vi "rsidr_core_global.vi"() -> ()   [LabVIEW 2020, in "Rohde&Schwarz CMWXP NR FR1 Measurement.lvlib"] (continued)
measured list mode segments.\n\nReturn values:  \n<Reliability>\n decimal\n\n<TimingError>\n float\nComma-separated list of values, one per measured segment\nDefault unit:  Ts (basic time unit)\n\nAvailable Repeated Capabilities:\ninstance: i0, i1, i2, i3, i4, i5, i6, i7, i8, i9, i10, i11, i12, i13, i14, i15, i16, i17, i18, i19, i20, i21, i22, i23, i24, i25, i26, i27, i28, i29, i30, i31, i32\r\n\nRemote-control command(s):\nFETCh:NRSub:MEAS<i>:MEValuation:LIST:MODulation:TERRor:SDEViation?"}, {"Level"=5, "Class Only"=FALSE, "Identifier"="RSCMWXPNRFR1M_ATTR_QUERY_MULTI_EVAL_MEAS_LIST_TERR_CURRENT_LIMIT_CHECK_RESULTS", "Descriptive Name"="Query Multi Eval Meas List TERR Current Limit Check Results", "Data Type"=enum."RawString", "Command"="CALC:NRS:MEAS{instance}:MEV:LIST:MOD:TERR:CURR?", "Access"=enum."Read Only", "Range Table"="", "Read Callback"="", "Write Callback"="", "Range Callback"="", "Check Callback"="", "Rngtable Callback"="", "Coerce Callback"="", "Supported Models"="", "Instrument Options"="", "Check Status Callback"="", "Flags"=0, "Help"="Return transmit time error limit check results for all measured list mode segments.\n\nReturn values:  \n<Reliability>\n decimal\n\n<TimingErrorLimCheck>\n limit check result\nComma-separated list of values, one per measured segment\n\nAvailable Repeated Capabilities:\ninstance: i0, i1, i2, i3, i4, i5, i6, i7, i8, i9, i10, i11, i12, i13, i14, i15, i16, i17, i18, i19, i20, i21, i22, i23, i24, i25, i26, i27, i28, i29, i30, i31, i32\r\n\nRemote-control command(s):\nCALCulate:NRSub:MEAS<i>:MEValuation:LIST:MODulation:TERRor:CURRent?"}, {"Level"=5, "Class Only"=FALSE, "Identifier"="RSCMWXPNRFR1M_ATTR_QUERY_MULTI_EVAL_MEAS_LIST_TERR_AVERAGE_LIMIT_CHECK_RESULTS", "Descriptive Name"="Query Multi Eval Meas List TERR Average Limit Check Results", "Data Type"=enum."RawString", "Command"="CALC:NRS:MEAS{instance}:MEV:LIST:MOD:TERR:AVER?", "Access"=enum."Read Only", "Range Table"="", "Read Callback"="", "Write Callback"="", "Range Callback"="", "Check Callback"="", "Rngtable Callback"="", "Coerce Callback"="", "Supported Models"="", "Instrument Options"="", "Check Status Callback"="", "Flags"=0, "Help"="Return average transmit time error limit check results for all measured list mode segments.\n\nReturn values:  \n<Reliability>\n decimal\n\n<TimingErrorLimCheck>\n limit check result\nComma-separated list of values, one per measured segment\n\nAvailable Repeated Capabilities:\ninstance: i0, i1, i2, i3, i4, i5, i6, i7, i8, i9, i10, i11, i12, i13, i14, i15, i16, i17, i18, i19, i20, i21, i22, i23, i24, i25, i26, i27, i28, i29, i30, i31, i32\r\n\nRemote-control command(s):\nCALCulate:NRSub:MEAS<i>:MEValuation:LIST:MODulation:TERRor:AVERage?"}, {"Level"=5, "Class Only"=FALSE, "Identifier"="RSCMWXPNRFR1M_ATTR_QUERY_MULTI_EVAL_MEAS_LIST_TERR_EXTREME_LIMIT_CHECK_RESULTS", "Descriptive Name"="Query Multi Eval Meas List TERR Extreme Limit Check Results", "Data Type"=enum."RawString", "Command"="CALC:NRS:MEAS{instance}:MEV:LIST:MOD:TERR:EXTR?", "Access"=enum."Read Only", "Range Table"="", "Read Callback"="", "Write Callback"="", "Range Callback"="", "Check Callback"="", "Rngtable Callback"="", "Coerce Callback"="", "Supported Models"="", "Instrument Options"="", "Check Status Callback"="", "Flags"=0, "Help"="Return extreme transmit time error limit check results for all measured list mode segments.\n\nReturn values:  \n<Reliability>\n decimal\n\n<TimingErrorLimCheck>\n limit check result\nComma-separated list of values, one per measured segment\n\nAvailable Repeated Capabilities:\ninstance: i0, i1, i2, i3, i4, i5, i6, i7, i8, i9, i10, i11, i12, i13, i14, i15, i16, i17, i18, i19, i20, i21, i22, i23, i24, i25, i26, i27, i28, i29, i30, i31, i32\r\n\nRemote-control command(s):\nCALCulate:NRSub:MEAS<i>:MEValuation:LIST:MODulation:TERRor:EXTReme?"}, {"Level"=4, "Class Only"=TRUE, "Identifier"="", "Descriptive Name"="User Equipment Power", "Data Type"=enum."ViInt32", "Command"="", "Access"=enum."Read Only", "Range Table"="", "Read Callback"="", "Write Callback"="", "Range Callback"="", "Check Callback"="", "Rngtable Callback"="", "Coerce Callback"="", "Supported Models"="", "Instrument Options"="", "Check Status Callback"="", "Flags"=0, "Help"="The attributes in this class return user equipment power results for all measured segments. The number of returned results depends on the number of measured segments."}, {"Level"=5, "Class Only"=FALSE, "Identifier"="RSCMWXPNRFR1M_ATTR_FETCH_MULTI_EVAL_MEAS_LIST_TPOWER_CURRENT_RESULTS", "Descriptive Name"="Fetch Multi Eval Meas List TPower Current Results", "Data Type"=enum."RawString", "Command"="FETC:NRS:MEAS{instance}:MEV:LIST:MOD:TPOW:CURR?", "Access"=enum."Read Only", "Range Table"="", "Read Callback"="", "Write Callback"="", "Range Callback"="", "Check Callback"="", "Rngtable Callback"="", "Coerce Callback"="", "Supported Models"="", "Instrument Options"="", "Check Status Callback"="", "Flags"=0, "Help"="Return user equipment power values for all measured list mode segments.\n\nReturn values:  \n<Reliability>\n decimal\n\n<TXpower>\n float\nComma-separated list of values, one per measured segment\nDefault unit:  dBm\n\nAvailable Repeated Capabilities:\ninstance: i0, i1, i2, i3, i4, i5, i6, i7, i8, i9, i10, i11, i12, i13, i14, i15, i16, i17, i18, i19, i20, i21, i22, i23, i24, i25, i26, i27, i28, i29, i30, i31, i32\r\n\nRemote-control command(s):\nFETCh:NRSub:MEAS<i>:MEValuation:LIST:MODulation:TPOWer:CURRent?"}, {"Level"=5, "Class Only"=FALSE, "Identifier"="RSCMWXPNRFR1M_ATTR_FETCH_MULTI_EVAL_MEAS_LIST_TPOWER_AVERAGE_RESULTS", "Descriptive Name"="Fetch Multi Eval Meas List TPower Average Results", "Data Type"=enum."RawString", "Command"="FETC:NRS:MEAS{instance}:MEV:LIST:MOD:TPOW:AVER?", "Access"=enum."Read Only", "Range Table"="", "Read Callback"="", "Write Callback"="", "Range Callback"="", "Check Callback"="", "Rngtable Callback"="", "Coerce Callback"="", "Supported Models"="", "Instrument Options"="", "Check Status Callback"="", "Flags"=0, "Help"="Return everage user equipment power values for all measured list mode segments.\n\nReturn values:  \n<Reliability>\n decimal\n\n<TXpower>\n float\nComma-separated list of values, one per measured segment\nDefault unit:  dBm\n\nAvailable Repeated Capabilities:\ninstance: i0, i1, i2, i3, i4, i5, i6, i7, i8, i9, i10, i11, i12, i13, i14, i15, i16, i17, i18, i19, i20, i21, i22, i23, i24, i25, i26, i27, i28, i29, i30, i31, i32\r\n\nRemote-control command(s):\nFETCh:NRSub:MEAS<i>:MEValuation:LIST:MODulation:TPOWer:AVERage?"}, {"Level"=5, "Class Only"=FALSE, "Identifier"="RSCMWXPNRFR1M_ATTR_FETCH_MULTI_EVAL_MEAS_LIST_TPOWER_STANDARD_DEVIATION_RESULTS", "Descriptive Name"="Fetch Multi Eval Meas List TPower Standard Deviation Results", "Data Type"=enum."RawString", "Command"="FETC:NRS:MEAS{instance}:MEV:LIST:MOD:TPOW:SDEV?", "Access"=enum."Read Only", "Range Table"="", "Read Callback"="", "Write Callback"="", "Range Callback"="", "Check Callback"="", "Rngtable Callback"="", "Coerce Callback"="", "Supported Models"="", "Instrument Options"="", "Check Status Callback"="", "Flags"=0, "Help"="Return standard deviation user equipment power values for all measured list mode segments.\n\nReturn values:  \n<Reliability>\n decimal\n\n<TXpower>\n float\nComma-separated list of values, one per measured segment\nDefault unit:  dBm\n\nAvailable Repeated Capabilities:\ninstance: i0, i1, i2, i3, i4, i5, i6, i7, i8, i9, i10, i11, i12, i13, i14, i15, i16, i17, i18, i19, i20, i21, i22, i23, i24, i25, i26, i27, i28, i29, i30, i31, i32\r\n\nRemote-control command(s):\nFETCh:NRSub:MEAS<i>:MEValuation:LIST:MODulation:TPOWer:SDEViation?"}, {"Level"=5, "Class Only"=FALSE, "Identifier"="RSCMWXPNRFR1M_ATTR_FETCH_MULTI_EVAL_MEAS_LIST_TPOWER_MAXIMUM_RESULTS", "Descriptive Name"="Fetch Multi Eval Meas List TPower Maximum Results", "Data Type"=enum."RawString", "Command"="FETC:NRS:MEAS{instance}:MEV:LIST:MOD:TPOW:MAX?", "Access"=enum."Read Only", "Range Table"="", "Read Callback"="", "Write Callback"="", "Range Callback"="", "Check Callback"="", "Rngtable Callback"="", "Coerce Callback"="", "Supported Models"="", "Instrument Options"="", "Check Status Callback"="", "Flags"=0, "Help"="Return maximum user equipment power values for all measured list mode segments.\n\nReturn values:  \n<Reliability>\n decimal\n\n<TXpower>\n float\nComma-separated list of values, one per measured segment\nDefault unit:  dBm\n\nAvailable Repeated Capabilities:\ninstance: i0, i1, i2, i3, i4, i5, i6, i7, i8, i9, i10, i11, i12, i13, i14, i15, i16, i17, i18, i19, i20, i21, i22, i23, i24, i25, i26, i27, i28, i29, i30, i31, i32\r\n\nRemote-control command(s):\nFETCh:NRSub:MEAS<i>:MEValuation:LIST:MODulation:TPOWer:MAXimum?"}, {"Level"=5, "Class Only"=FALSE, "Identifier"="RSCMWXPNRFR1M_ATTR_FETCH_MULTI_EVAL_MEAS_LIST_TPOWER_MINIMUM_RESULTS", "Descriptive Name"="Fetch Multi Eval Meas List TPower Minimum Results", "Data Type"=enum."RawString", "Command"="FETC:NRS:MEAS{instance}:MEV:LIST:MOD:TPOW:MIN?", "Access"=enum."Read Only", "Range Table"="", "Read Callback"="", "Write Callback"="", "Range Callback"="", "Check Callback"="", "Rngtable Callback"="", "Coerce Callback"="", "Supported Models"="", "Instrument Options"="", "Check Status Callback"="", "Flags"=0, "Help"="Return minimum user equipment power values for all measured list mode segments.\n\nReturn values:  \n<Reliability>\n decimal\n\n<TXpower>\n float\nComma-separated list of values, one per measured segment\nDefault unit:  dBm\n\nAvailable Repeated Capabilities:\ninstance: i0, i1, i2, i3, i4, i5, i6, i7, i8, i9, i10, i11, i12, i13, i14, i15, i16, i17, i18, i19, i20, i21, i22, i23, i24, i25, i26, i27, i28, i29, i30, i31, i32\r\n\nRemote-control command(s):\nFETCh:NRSub:MEAS<i>:MEValuation:LIST:MODulation:TPOWer:MINimum?"}, {"Level"=5, "Class Only"=FALSE, "Identifier"="RSCMWXPNRFR1M_ATTR_QUERY_MULTI_EVAL_MEAS_LIST_TPOWER_CURRENT_LIMIT_CHECK_RESULTS", "Descriptive Name"="Query Multi Eval Meas List TPower Current Limit Check Results", "Data Type"=enum."RawString", "Command"="CALC:NRS:MEAS{instance}:MEV:LIST:MOD:TPOW:CURR?", "Access"=enum."Read Only", "Range Table"="", "Read Callback"="", "Write Callback"="", "Range Callback"="", "Check Callback"="", "Rngtable Callback"="", "Coerce Callback"="", "Supported Models"="", "Instrument Options"="", "Check Status Callback"="", "Flags"=0, "Help"="Return user equipment power limit check results for all measured list mode segments.\n\nReturn values:  \n<Reliability>\n decimal\n\n<TXpowerLimCheck>\n limit check result\nComma-separated list of values, one per measured segment\n\nAvailable Repeated Capabilities:\ninstance: i0, i1, i2, i3, i4, i5, i6, i7, i8, i9, i10, i11, i12, i13, i14, i15, i16, i17, i18, i19, i20, i21, i22, i23, i24, i25, i26, i27, i28, i29, i30, i31, i32\r\n\nRemote-control command(s):\nCALCulate:NRSub:MEAS<i>:MEValuation:LIST:MODulation:TPOWer:CURRent?"}, {"Level"=5, "Class Only"=FALSE, "Identifier"="RSCMWXPNRFR1M_ATTR_QUERY_MULTI_EVAL_MEAS_LIST_TPOWER_AVERAGE_LIMIT_CHECK_RESULTS", "Descriptive Name"="Query Multi Eval Meas List TPower Average Limit Check Results", "Data Type"=enum."RawString", "Command"="CALC:NRS:MEAS{instance}:MEV:LIST:MOD:TPOW:AVER?", "Access"=enum."Read Only", "Range Table"="", "Read Callback"="", "Write Callback"="", "Range Callback"="", "Check Callback"="", "Rngtable Callback"="", "Coerce Callback"="", "Supported Models"="", "Instrument Options"="", "Check Status Callback"="", "Flags"=0, "Help"="Return average user equipment power limit check results for all measured list mode segments.\n\nReturn values:  \n<Reliability>\n decimal\n\n<TXpowerLimCheck>\n limit check result\nComma-separated list of values, one per measured segment\n\nAvailable Repeated Capabilities:\ninstance: i0, i1, i2, i3, i4, i5, i6, i7, i8, i9, i10, i11, i12, i13, i14, i15, i16, i17, i18, i19, i20, i21, i22, i23, i24, i25, i26, i27, i28, i29, i30, i31, i32\r\n\nRemote-control command(s):\nCALCulate:NRSub:MEAS<i>:MEValuation:LIST:MODulation:TPOWer:AVERage?"}, {"Level"=5, "Class Only"=FALSE, "Identifier"="RSCMWXPNRFR1M_ATTR_QUERY_MULTI_EVAL_MEAS_LIST_TPOWER_MAXIMUM_LIMIT_CHECK_RESULTS", "Descriptive Name"="Query Multi Eval Meas List TPower Maximum Limit Check Results", "Data Type"=enum."RawString", "Command"="CALC:NRS:MEAS{instance}:MEV:LIST:MOD:TPOW:MAX?", "Access"=enum."Read Only", "Range Table"="", "Read Callback"="", "Write Callback"="", "Range Callback"="", "Check Callback"="", "Rngtable Callback"="", "Coerce Callback"="", "Supported Models"="", "Instrument Options"="", "Check Status Callback"="", "Flags"=0, "Help"="Return maximum user equipment power limit check results for all measured list mode segments.\n\nReturn values:  \n<Reliability>\n decimal\n\n<TXpowerLimCheck>\n limit check result\nComma-separated list of values, one per measured segment\n\nAvailable Repeated Capabilities:\ninstance: i0, i1, i2, i3, i4, i5, i6, i7, i8, i9, i10, i11, i12, i13, i14, i15, i16, i17, i18, i19, i20, i21, i22, i23, i24, i25, i26, i27, i28, i29, i30, i31, i32\r\n\nRemote-control command(s):\nCALCulate:NRSub:MEAS<i>:MEValuation:LIST:MODulation:TPOWer:MAXimum?"}, {"Level"=5, "Class Only"=FALSE, "Identifier"="RSCMWXPNRFR1M_ATTR_QUERY_MULTI_EVAL_MEAS_LIST_TPOWER_MINIMUM_LIMIT_CHECK_RESULTS", "Descriptive Name"="Query Multi Eval Meas List TPower Minimum Limit Check Results", "Data Type"=enum."RawString", "Command"="CALC:NRS:MEAS{instance}:MEV:LIST:MOD:TPOW:MIN?", "Access"=enum."Read Only", "Range Table"="", "Read Callback"="", "Write Callback"="", "Range Callback"="", "Check Callback"="", "Rngtable Callback"="", "Coerce Callback"="", "Supported Models"="", "Instrument Options"="", "Check Status Callback"="", "Flags"=0, "Help"="Return minimum user equipment power limit check results for all measured list mode segments.\n\nReturn values:  \n<Reliability>\n decimal\n\n<TXpowerLimCheck>\n limit check result\nComma-separated list of values, one per measured segment\n\nAvailable Repeated Capabilities:\ninstance: i0, i1, i2, i3, i4, i5, i6, i7, i8, i9, i10, i11, i12, i13, i14, i15, i16, i17, i18, i19, i20, i21, i22, i23, i24, i25, i26, i27, i28, i29, i30, i31, i32\r\n\nRemote-control command(s):\nCALCulate:NRSub:MEAS<i>:MEValuation:LIST:MODulation:TPOWer:MINimum?"}, {"Level"=4, "Class Only"=TRUE, "Identifier"="", "Descriptive Name"="Spectrum Emission Mask", "Data Type"=enum."ViInt32", "Command"="", "Access"=enum."Read Only", "Range Table"="", "Read Callback"="", "Write Callback"="", "Range Callback"="", "Check Callback"="", "Rngtable Callback"="", "Coerce Callback"="", "Supported Models"="", "Instrument Options"="", "Check Status Callback"="", "Flags"=0, "Help"="The attributes in this class return spectrum emission mask results for all measured segments. The number of returned results depends on the number of measured segments."}, {"Level"=5, "Class Only"=FALSE, "Identifier"="RSCMWXPNRFR1M_ATTR_FETCH_MULTI_EVAL_MEAS_LIST_SEM_OBW_CURRENT_RESULTS", "Descriptive Name"="Fetch Multi Eval Meas List SEM OBW Current Results", "Data Type"=enum."RawString", "Command"="FETC:NRS:MEAS{instance}:MEV:LIST:SEM:OBW:CURR?", "Access"=enum."Read Only", "Range Table"="", "Read Callback"="", "Write Callback"="", "Range Callback"="", "Check Callback"="", "Rngtable Callback"="", "Coerce Callback"="", "Supported Models"="", "Instrument Options"="", "Check Status Callback"="", "Flags"=0, "Help"="Return the occupied bandwidth for all measured list mode segments.\n\nReturn values:  \n<Reliability>\n decimal\n\n<OBW>\n float\nComma-separated list of values, one per measured segment\nDefault unit:  Hz\n\nAvailable Repeated Capabilities:\ninstance: i0, i1, i2, i3, i4, i5, i6, i7, i8, i9, i10, i11, i12, i13, i14, i15, i16, i17, i18, i19, i20, i21, i22, i23, i24, i25, i26, i27, i28, i29, i30, i31, i32\r\n\nRemote-control command(s):\nFETCh:NRSub:MEAS<i>:MEValuation:LIST:SEMask:OBW:CURRent?"}, {"Level"=5, "Class Only"=FALSE, "Identifier"="RSCMWXPNRFR1M_ATTR_FETCH_MULTI_EVAL_MEAS_LIST_SEM_OBW_AVERAGE_RESULTS", "Descriptive Name"="Fetch Multi Eval Meas List SEM OBW Average Results", "Data Type"=enum."RawString", "Command"="FETC:NRS:MEAS{instance}:MEV:LIST:SEM:OBW:AVER?", "Access"=enum."Read Only", "Range Table"="", "Read Callback"="", "Write Callback"="", "Range Callback"="", "Check Callback"="", "Rngtable Callback"="", "Coerce Callback"="", "Supported Models"="", "Instrument Options"="", "Check Status Callback"="", "Flags"=0, "Help"="Return average the occupied bandwidth for all measured list mode segments.\n\nReturn values:  \n<Reliability>\n decimal\n\n<OBW>\n float\nComma-separated list of values, one per measured segment\nDefault unit:  Hz\n\nAvailable Repeated Capabilities:\ninstance: i0, i1, i2, i3, i4, i5, i6, i7, i8, i9, i10, i11, i12, i13, i14, i15, i16, i17, i18, i19, i20, i21, i22, i23, i24, i25, i26, i27, i28, i29, i30, i31, i32\r\n\nRemote-control command(s):\nFETCh:NRSub:MEAS<i>:MEValuation:LIST:SEMask:OBW:AVERage?"}, {"Level"=5, "Class Only"=FALSE, "Identifier"="RSCMWXPNRFR1M_ATTR_FETCH_MULTI_EVAL_MEAS_LIST_SEM_OBW_EXTREME_RESULTS", "Descriptive Name"="Fetch Multi Eval Meas List SEM OBW Extreme Results", "Data Type"=enum."RawString", "Command"="FETC:NRS:MEAS{instance}:MEV:LIST:SEM:OBW:EXTR?", "Access"=enum."Read Only", "Range Table"="", "Read Callback"="", "Write Callback"="", "Range Callback"="", "Check Callback"="", "Rngtable Callback"="", "Coerce Callback"="", "Supported Models"="", "Instrument Options"="", "Check Status Callback"="", "Flags"=0, "Help"="Return extreme the occupied bandwidth for all measured list mode segments.\n\nReturn values:  \n<Reliability>\n decimal\n\n<OBW>\n float\nComma-separated list of values, one per measured segment\nDefault unit:  Hz\n\nAvailable Repeated Capabilities:\ninstance: i0, i1, i2, i3, i4, i5, i6, i7, i8, i9, i10, i11, i12, i13, i14, i15, i16, i17, i18, i19, i20, i21, i22, i23, i24, i25, i26, i27, i28, i29, i30, i31, i32\r\n\nRemote-control command(s):\nFETCh:NRSub:MEAS<i>:MEValuation:LIST:SEMask:OBW:EXTReme?"}, {"Level"=5, "Class Only"=FALSE, "Identifier"="RSCMWXPNRFR1M_ATTR_FETCH_MULTI_EVAL_MEAS_LIST_SEM_OBW_STANDARD_DEVIATION_RESULTS", "Descriptive Name"="Fetch Multi Eval Meas List SEM OBW Standard Deviation Results", "Data Type"=enum."RawString", "Command"="FETC:NRS:MEAS{instance}:MEV:LIST:SEM:OBW:SDEV?", "Access"=enum."Read Only", "Range Table"="", "Read Callback"="", "Write Callback"="", "Range Callback"="", "Check Callback"="", "Rngtable Callback"="", "Coerce Callback"="", "Supported Models"="", "Instrument Options"="", "Check Status Callback"="", "Flags"=0, "Help"="Return standard deviation the occupied bandwidth for all measured list mode segments.\n\nReturn values:  \n<Reliability>\n decimal\n\n<OBW>\n float\nComma-separated list of values, one per measured segment\nDefault unit:  Hz\n\nAvailable Repeated Capabilities:\ninstance: i0, i1, i2, i3, i4, i5, i6, i7, i8, i9, i10, i11, i12, i13, i14, i15, i16, i17, i18, i19, i20, i21, i22, i23, i24, i25, i26, i27, i28, i29, i30, i31, i32\r\n\nRemote-control command(s):\nFETCh:NRSub:MEAS<i>:MEValuation:LIST:SEMask:OBW:SDEViation?"}, {"Level"=5, "Class Only"=FALSE, "Identifier"="RSCMWXPNRFR1M_ATTR_QUERY_MULTI_EVAL_MEAS_LIST_SEM_OBW_CURRENT_LIMIT_CHECK_RESULTS", "Descriptive Name"="Query Multi Eval Meas List SEM OBW Current Limit Check Results", "Data Type"=enum."RawString", "Command"="CALC:NRS:MEAS{instance}:MEV:LIST:SEM:OBW:CURR?", "Access"=enum."Read Only", "Range Table"="", "Read Callback"="", "Write Callback"="", "Range Callback"="", "Check Callback"="", "Rngtable Callback"="", "Coerce Callback"="", "Supported Models"="", "Instrument Options"="", "Check Status Callback"="", "Flags"=0, "Help"="Return the occupied bandwidth limit check results for all measured list mode segments.\n\nReturn values:  \n<Reliability>\n decimal\n\n<OBWLimCheck>\n limit check result\nComma-separated list of values, one per measured segment\n\nAvailable Repeated Capabilities:\ninstance: i0, i1, i2, i3, i4, i5, i6, i7, i8, i9, i10, i11, i12, i13, i14, i15, i16, i17, i18, i19, i20, i21, i22, i23, i24, i25, i26, i27, i28, i29, i30, i31, i32\r\n\nRemote-control command(s):\nCALCulate:NRSub:MEAS<i>:MEValuation:LIST:SEMask:OBW:CURRent?"}, {"Level"=5, "Class Only"=FALSE, "Identifier"="RSCMWXPNRFR1M_ATTR_QUERY_MULTI_EVAL_MEAS_LIST_SEM_OBW_AVERAGE_LIMIT_CHECK_RESULTS", "Descriptive Name"="Query Multi Eval Meas List SEM OBW Average Limit Check Results", "Data Type"=enum."RawString", "Command"="CALC:NRS:MEAS{instance}:MEV:LIST:SEM:OBW:AVER?", "Access"=enum."Read Only", "Range Table"="", "Read Callback"="", "Write Callback"="", "Range Callback"="", "Check Callback"="", "Rngtable Callback"="", "Coerce Callback"="", "Supported Models"="", "Instrument Options"="", "Check Status Callback"="", "Flags"=0, "Help"="Return the average occupied bandwidth limit check results for all measured list mode segments.\n\nReturn values:  \n<Reliability>\n decimal\n\n<OBWLimCheck>\n limit check result\nComma-separated list of values, one per measured segment\n\nAvailable Repeated Capabilities:\ninstance: i0, i1, i2, i3, i4, i5, i6, i7, i8, i9, i10, i11, i12, i13, i14, i15, i16, i17, i18, i19, i20, i21, i22, i23, i24, i25, i26, i27, i28, i29, i30, i31, i32\r\n\nRemote-control command(s):\nCALCulate:NRSub:MEAS<i>:MEValuation:LIST:SEMask:OBW:AVERage?"}, {"Level"=5, "Class Only"=FALSE, "Identifier"="RSCMWXPNRFR1M_ATTR_QUERY_MULTI_EVAL_MEAS_LIST_SEM_OBW_EXTREME_LIMIT_CHECK_RESULTS", "Descriptive Name"="Query Multi Eval Meas List SEM OBW Extreme Limit Check Results", "Data Type"=enum."RawString", "Command"="CALC:NRS:MEAS{instance}:MEV:LIST:SEM:OBW:EXTR?", "Access"=enum."Read Only", "Range Table"="", "Read Callback"="", "Write Callback"="", "Range Callback"="", "Check Callback"="", "Rngtable Callback"="", "Coerce Callback"="", "Supported Models"="", "Instrument Options"="", "Check Status Callback"="", "Flags"=0, "Help"="Return the extreme occupied bandwidth limit check results for all measured list mode segments.\n\nReturn values:  \n<Reliability>\n decimal\n\n<OBWLimCheck>\n limit check result\nComma-separated list of values, one per measured segment\n\nAvailable Repeated Capabilities:\ninstance: i0, i1, i2, i3, i4, i5, i6, i7, i8, i9, i10, i11, i12, i13, i14, i15, i16, i17, i18, i19, i20, i21, i22, i23, i24, i25, i26, i27, i28, i29, i30, i31, i32\r\n\nRemote-control command(s):\nCALCulate:NRSub:MEAS<i>:MEValuation:LIST:SEMask:OBW:EXTReme?"}, {"Level"=5, "Class Only"=FALSE, "Identifier"="RSCMWXPNRFR1M_ATTR_FETCH_MULTI_EVAL_MEAS_LIST_SEM_TX_POWER_CURRENT_RESULTS", "Descriptive Name"="Fetch Multi Eval Meas List SEM TX Power Current Results", "Data Type"=enum."RawString", "Command"="FETC:NRS:MEAS{instance}:MEV:LIST:SEM:TXP:CURR?", "Access"=enum."Read Only", "Range Table"="", "Read Callback"="", "Write Callback"="", "Range Callback"="", "Check Callback"="", "Rngtable Callback"="", "Coerce Callback"="", "Supported Models"="", "Instrument Options"="", "Check Status Callback"="", "Flags"=0, "Help"="Return the total TX power in the slot for all measured list mode segments.\n\nReturn values:  \n<Reliability>\n decimal\n\n<TXpower>\n float\nComma-separated list of values, one per measured segment\nDefault unit:  dBm\n\nAvailable Repeated Capabilities:\ninstance: i0, i1, i2, i3, i4, i5, i6, i7, i8, i9, i10, i11, i12, i13, i14, i15, i16, i17, i18, i19, i20, i21, i22, i23, i24, i25, i26, i27, i28, i29, i30, i31, i32\r\n\nRemote-control command(s):\nFETCh:NRSub:MEAS<i>:MEValuation:LIST:SEMask:TXPower:CURRent?"}, {"Level"=5, "Class Only"=FALSE, "Identifier"="RSCMWXPNRFR1M_ATTR_FETCH_MULTI_EVAL_MEAS_LIST_SEM_TX_POWER_AVERAGE_RESULTS", "Descriptive Name"="Fetch Multi Eval Meas List SEM TX Power Average Results", "Data Type"=enum."RawString", "Command"="FETC:NRS:MEAS{instance}:MEV:LIST:SEM:TXP:AVER?", "Access"=enum."Read Only", "Range Table"="", "Read Callback"="", "Write Callback"="", "Range Callback"="", "Check Callback"="", "Rngtable Callback"="", "Coerce Callback"="", "Supported Models"="", "Instrument Options"="", "Check Status Callback"="", "Flags"=0, "Help"="Return the average total TX power in the slot for all measured list mode segments.\n\nReturn values:  \n<Reliability>\n decimal\n\n<TXpower>\n float\nComma-separated list of values, one per measured segment\nDefault unit:  dBm\n\nAvailable Repeated Capabilities:\ninstance: i0, i1, i2, i3, i4, i5, i6, i7, i8, i9, i10, i11, i12, i13, i14, i15, i16, i17, i18, i19, i20, i21, i22, i23, i24, i25, i26, i27, i28, i29, i30, i31, i32\r\n\nRemote-control command(s):\nFETCh:NRSub:MEAS<i>:MEValuation:LIST:SEMask:TXPower:AVERage?"}, {"Level"=5, "Class Only"=FALSE, "Identifier"="RSCMWXPNRFR1M_ATTR_FETCH_MULTI_EVAL_MEAS_LIST_SEM_TX_POWER_STANDARD_DEVIATION_RESULTS", "Descriptive Name"="Fetch Multi Eval Meas List SEM TX Power Standard Deviation Results", "Data Type"=enum."RawString", "Command"="FETC:NRS:MEAS{instance}:MEV:LIST:SEM:TXP:SDEV?", "Access"=enum."Read Only", "Range Table"="", "Read Callback"="", "Write Callback"="", "Range Callback"="", "Check Callback"="", "Rngtable Callback"="", "Coerce Callback"="", "Supported Models"="", "Instrument Options"="", "Check Status Callback"="", "Flags"=0, "Help"="Return the standard deviation total TX power in the slot for all measured list mode segments.\n\nReturn values:  \n<Reliability>\n decimal\n\n<TXpower>\n float\nComma-separated list of values, one per measured segment\nDefault unit:  dBm\n\nAvailable Repeated Capabilities:\ninstance: i0, i1, i2, i3, i4, i5, i6, i7, i8, i9, i10, i11, i12, i13, i14, i15, i16, i17, i18, i19, i20, i21, i22, i23, i24, i25, i26, i27, i28, i29, i30, i31, i32\r\n\nRemote-control command(s):\nFETCh:NRSub:MEAS<i>:MEValuation:LIST:SEMask:TXPower:SDEViation?"}, {"Level"=5, "Class Only"=FALSE, "Identifier"="RSCMWXPNRFR1M_ATTR_FETCH_MULTI_EVAL_MEAS_LIST_SEM_TX_POWER_MAXIMUM_RESULTS", "Descriptive Name"="Fetch Multi Eval Meas List SEM TX Power Maximum Results", "Data Type"=enum."RawString", "Command"="FETC:NRS:MEAS{instance}:MEV:LIST:SEM:TXP:MAX?", "Access"=enum."Read Only", "Range Table"="", "Read Callback"="", "Write Callback"="", "Range Callback"="", "Check Callback"="", "Rngtable Callback"="", "Coerce Callback"="", "Supported Models"="", "Instrument Options"="", "Check Status Callback"="", "Flags"=0, "Help"="Return the maximum total TX power in the slot for all measured list mode segments.\n\nReturn values:  \n<Reliability>\n decimal\n\n<TXpower>\n float\nComma-separated list of values, one per measured segment\nDefault unit:  dBm\n\nAvailable Repeated Capabilities:\ninstance: i0, i1, i2, i3, i4, i5, i6, i7, i8, i9, i10, i11, i12, i13, i14, i15, i16, i17, i18, i19, i20, i21, i22, i23, i24, i25, i26, i27, i28, i29, i30, i31, i32\r\n\nRemote-control command(s):\nFETCh:NRSub:MEAS<i>:MEValuation:LIST:SEMask:TXPower:MAXimum?"}, {"Level"=5, "Class Only"=FALSE, "Identifier"="RSCMWXPNRFR1M_ATTR_FETCH_MULTI_EVAL_MEAS_LIST_SEM_TX_POWER_MINIMUM_RESULTS", "Descriptive Name"="Fetch Multi Eval Meas List SEM TX Power Minimum Results", "Data Type"=enum."RawString", "Command"="FETC:NRS:MEAS{instance}:MEV:LIST:SEM:TXP:MIN?", "Access"=enum."Read Only", "Range Table"="", "Read Callback"="", "Write Callback"="", "Range Callback"="", "Check Callback"="", "Rngtable Callback"="", "Coerce Callback"="", "Supported Models"="", "Instrument Options"="", "Check Status Callback"="", "Flags"=0, "Help"="Return the minimum total TX power in the slot for all measured list mode segments.\n\nReturn values:  \n<Reliability>\n decimal\n\n<TXpower>\n float\nComma-separated list of values, one per measured segment\nDefault unit:  dBm\n\nAvailable Repeated Capabilities:\ninstance: i0, i1, i2, i3, i4, i5, i6, i7, i8, i9, i10, i11, i12, i13, i14, i15, i16, i17, i18, i19, i20, i21, i22, i23, i24, i25, i26, i27, i28, i29, i30, i31, i32\r\n\nRemote-control command(s):\nFETCh:NRSub:MEAS<i>:MEValuation:LIST:SEMask:TXPower:MINimum?"}, {"Level"=5, "Class Only"=FALSE, "Identifier"="RSCMWXPNRFR1M_ATTR_QUERY_MULTI_EVAL_MEAS_LIST_SEM_TX_POWER_CURRENT_LIMIT_CHECK_RESULTS", "Descriptive Name"="Query Multi Eval Meas List SEM TX Power Current Limit Check Results", "Data Type"=enum."RawString", "Command"="CALC:NRS:MEAS{instance}:MEV:LIST:SEM:TXP:CURR?", "Access"=enum."Read Only", "Range Table"="", "Read Callback"="", "Write Callback"="", "Range Callback"="", "Check Callback"="", "Rngtable Callback"="", "Coerce Callback"="", "Supported Models"="", "Instrument Options"="", "Check Status Callback"="", "Flags"=0, "Help"="Return the total TX power limit check results in the slot for all measured list mode segments.\n\nReturn values:  \n<Reliability>\n decimal\n\n<TXpowerLimCheck>\n limit check result\nComma-separated list of values, one per measured segment\n\nAvailable Repeated Capabilities:\ninstance: i0, i1, i2, i3, i4, i5, i6, i7, i8, i9, i10, i11, i12, i13, i14, i15, i16, i17, i18, i19, i20, i21, i22, i23, i24, i25, i26, i27, i28, i29, i30, i31, i32\r\n\nRemote-control command(s):\nCALCulate:NRSub:MEAS<i>:MEValuation:LIST:SEMask:TXPower:CURRent?"}, {"Level"=5, "Class Only"=FALSE, "Identifier"="RSCMWXPNRFR1M_ATTR_QUERY_MULTI_EVAL_MEAS_LIST_SEM_TX_POWER_AVERAGE_LIMIT_CHECK_RESULTS", "Descriptive Name"="Query Multi Eval Meas List SEM TX Power Average Limit Check Results", "Data Type"=enum."RawString", "Command"="CALC:NRS:MEAS{instance}:MEV:LIST:SEM:TXP:AVER?", "Access"=enum."Read Only", "Range Table"="", "Read Callback"="", "Write Callback"="", "Range Callback"="", "Check Callback"="", "Rngtable Callback"="", "Coerce Callback"="", "Supported Models"="", "Instrument Options"="", "Check Status Callback"="", "Flags"=0, "Help"="Return the average total TX power limit check results in the slot for all measured list mode segments.\n\nReturn values:  \n<Reliability>\n decimal\n\n<TXpowerLimCheck>\n limit check result\nComma-separated list of values, one per measured segment\n\nAvailable Repeated Capabilities:\ninstance: i0, i1, i2, i3, i4, i5, i6, i7, i8, i9, i10, i11, i12, i13, i14, i15, i16, i17, i18, i19, i20, i21, i22, i23, i24, i25, i26, i27, i28, i29, i30, i31, i32\r\n\nRemote-control command(s):\nCALCulate:NRSub:MEAS<i>:MEValuation:LIST:SEMask:TXPower:AVERage?"}, {"Level"=5, "Class Only"=FALSE, "Identifier"="RSCMWXPNRFR1M_ATTR_QUERY_MULTI_EVAL_MEAS_LIST_SEM_TX_POWER_MAXIMUM_LIMIT_CHECK_RESULTS", "Descriptive Name"="Query Multi Eval Meas List SEM TX Power Maximum Limit Check Results", "Data Type"=enum."RawString", "Command"="CALC:NRS:MEAS{instance}:MEV:LIST:SEM:TXP:MAX?", "Access"=enum."Read Only", "Range Table"="", "Read Callback"="", "Write Callback"="", "Range Callback"="", "Check Callback"="", "Rngtable Callback"="", "Coerce Callback"="", "Supported Models"="", "Instrument Options"="", "Check Status Callback"="", "Flags"=0, "Help"="Return the maximum total TX power limit check results in the slot for all measured list mode segments.\n\nReturn values:  \n<Reliability>\n decimal\n\n<TXpowerLimCheck>\n limit check result\nComma-separated list of values, one per measured segment\n\nAvailable Repeated Capabilities:\ninstance: i0, i1, i2, i3, i4, i5, i6, i7, i8, i9, i10, i11, i12, i13, i14, i15, i16, i17, i18, i19, i20, i21, i22, i23, i24, i25, i26, i27, i28, i29, i30, i31, i32\r\n\nRemote-control command(s):\nCALCulate:NRSub:MEAS<i>:MEValuation:LIST:SEMask:TXPower:MAXimum?"}, {"Level"=5, "Class Only"=FALSE, "Identifier"="RSCMWXPNRFR1M_ATTR_QUERY_MULTI_EVAL_MEAS_LIST_SEM_TX_POWER_MINIMUM_LIMIT_CHECK_RESULTS", "Descriptive Name"="Query Multi Eval Meas List SEM TX Power Minimum Limit Check Results", "Data Type"=enum."RawString", "Command"="CALC:NRS:MEAS{instance}:MEV:LIST:SEM:TXP:MIN?", "Access"=enum."Read Only", "Range Table"="", "Read Callback"="", "Write Callback"="", "Range Callback"="", "Check Callback"="", "Rngtable Callback"="", "Coerce Callback"="", "Supported Models"="", "Instrument Options"="", "Check Status Callback"="", "Flags"=0, "Help"="Return the minimum total TX power limit check results in the slot for all measured list mode segments.\n\nReturn values:  \n<Reliability>\n decimal\n\n<TXpowerLimCheck>\n limit check result\nComma-separated list of values, one per measured segment\n\nAvailable Repeated Capabilities:\ninstance: i0, i1, i2, i3, i4, i5, i6, i7, i8, i9, i10, i11, i12, i13, i14, i15, i16, i17, i18, i19, i20, i21, i22, i23, i24, i25, i26, i27, i28, i29, i30, i31, i32\r\n\nRemote-control command(s):\nCALCulate:NRSub:MEAS<i>:MEValuation:LIST:SEMask:TXPower:MINimum?"}, {"Level"=5, "Class Only"=FALSE, "Identifier"="RSCMWXPNRFR1M_ATTR_FETCH_MULTI_EVAL_MEAS_LIST_SEM_DETECTED_ALLOCATION_RESULTS", "Descriptive Name"="Fetch Multi Eval Meas List SEM Detected Allocation Results", "Data Type"=enum."RawString", "Command"="FETC:NRS:MEAS{instance}:MEV:LIST:SEM:DALL?", "Access"=enum."Read Only", "Range Table"="", "Read Callback"="", "Write Callback"="", "Range Callback"="", "Check Callback"="", "Rngtable Callback"="", "Coerce Callback"="", "Supported Models"="", "Instrument Options"="", "Check Status Callback"="", "Flags"=0, "Help"="Return the detected allocation for all measured list mode segments. The result is determined from the last measured slot of the statistical length of a segment. The individual measurements provide identical detected allocation results when measuring the same slot. However different statistical lengths can be defined for the measurements so that the measured slots and returned results can differ.\n\nThe results are returned as pairs per segment: <Reliability>, {<NrResBlocks>, <OffsetResBlocks>}seg 1, {<NrResBlocks>, <OffsetResBlocks>}seg 2, ...\n\nReturn values:  \n<Reliability>\n decimal\n\n<NrResBlocks>\n decimal\nNumber of allocated resource blocks\n\n<OffsetResBlocks>\n decimal\nOffset of the first allocated resource block from the edge of the allocated UL transmission bandwidth\n\nAvailable Repeated Capabilities:\ninstance: i0, i1, i2, i3, i4, i5, i6, i7, i8, i9, i10, i11, i12, i13, i14, i15, i16, i17, i18, i19, i20, i21, i22, i23, i24, i25, i26, i27, i28, i29, i30, i31, i32\r\n\nRemote-control command(s):\nFETCh:NRSub:MEAS<i>:MEValuation:LIST:SEMask:DALLocation?"}, {"Level"=5, "Class Only"=TRUE, "Identifier"="", "Descriptive Name"="Area", "Data Type"=enum."ViInt32", "Command"="", "Access"=enum."Read Only", "Range Table"="", "Read Callback"="", "Write Callback"="", "Range Callback"="", "Check Callback"="", "Rngtable Callback"="", "Coerce Callback"="", "Supported Models"="", "Instrument Options"="", "Check Status Callback"="", "Flags"=0, "Help"="This class contains commands to fetch margin results for specific spectrum emission mask areas in list mode."}, {"Level"=6, "Class Only"=FALSE, "Identifier"="RSCMWXPNRFR1M_ATTR_FETCH_MULTI_EVAL_MEAS_LIST_SEM_MARGIN_AREA_POSITIVE_CURRENT_RESULTS", "Descriptive Name"="Fetch Multi Eval Meas List SEM Margin Area Positive Current Results", "Data Type"=enum."RawString", "Command"="FETC:NRS:MEAS{instance}:MEV:LIST:SEM:MARG:AREA{Area}:POS:CURR?", "Access"=enum."Read Only", "Range Table"="", "Read Callback"="", "Write Callback"="", "Range Callback"="", "Check Callback"="", "Rngtable Callback"="", "Coerce Callback"="", "Supported Models"="", "Instrument Options"="", "Check Status Callback"="", "Flags"=0, "Help"="Return spectrum emission mask margin positions for all measured list mode segments. The results of the current trace for positive offset frequencies are returned.\n\nThe results are returned as pairs per segment: <Reliability>, {<MarginPosX>, <MarginPosY>}seg 1, {<MarginPosX>, <MarginPosY>}seg 2, ...\n\nReturn values:  \n<Reliability>\n decimal\n\n<MarginPosX>\n float\nX-position of margin for selected area\nDefault unit:  Hz \n\n<MarginPosY>\n float\nY-position of margin for selected area\nDefault unit:  dB\n\nAvailable Repeated Capabilities:\ninstance: i0, i1, i2, i3, i4, i5, i6, i7, i8, i9, i10, i11, i12, i13, i14, i15, i16, i17, i18, i19, i20, i21, i22, i23, i24, i25, i26, i27, i28, i29, i30, i31, i32\r\nArea: a1, a2, a3, a4, a5, a6, a7, a8, a9, a10, a11, a12\r\n\nRemote-control command(s):\nFETCh:NRSub:MEAS<i>:MEValuation:LIST:SEMask:MARGin:AREA<no>:POSitiv:CURRent?"}, {"Level"=6, "Class Only"=FALSE, "Identifier"="RSCMWXPNRFR1M_ATTR_FETCH_MULTI_EVAL_MEAS_LIST_SEM_MARGIN_AREA_POSITIVE_AVERAGE_RESULTS", "Descriptive Name"="Fetch Multi Eval Meas List SEM Margin Area Positive Average Results", "Data Type"=enum."RawString", "Command"="FETC:NRS:MEAS{instance}:MEV:LIST:SEM:MARG:AREA{Area}:POS:AVER?", "Access"=enum."Read Only", "Range Table"="", "Read Callback"="", "Write Callback"="", "Range Callback"="", "Check Callback"="", "Rngtable Callback"="", "Coerce Callback"="", "Supported Models"="", "Instrument Options"="", "Check Status Callback"="", "Flags"=0, "Help"="Return spectrum emission mask margin positions for all measured list mode segments. The results of the average trace for positive offset frequencies are returned.\n\nThe results are returned as pairs per segment: <Reliability>, {<MarginPosX>, <MarginPosY>}seg 1, {<MarginPosX>, <MarginPosY>}seg 2, ...\n\nReturn values:  \n<Reliability>\n decimal\n\n<MarginPosX>\n float\nX-position of margin for selected area\nDefault unit:  Hz \n\n<MarginPosY>\n float\nY-position of margin for selected area\nDefault unit:  dB\n\nAvailable Repeated Capabilities:\ninstance: i0, i1, i2, i3, i4, i5, i6, i7, i8, i9, i10, i11, i12, i13, i14, i15, i16, i17, i18, i19, i20, i21, i22, i23, i24, i25, i26, i27, i28, i29, i30, i31, i32\r\nArea: a1, a2, a3, a4, a5, a6, a7, a8, a9, a10, a11, a12\r\n\nRemote-control command(s):\nFETCh:NRSub:MEAS<i>:MEValuation:LIST:SEMask:MARGin:AREA<no>:POSitiv:AVERage?"}, {"Level"=6, "Class Only"=FALSE, "Identifier"="RSCMWXPNRFR1M_ATTR_FETCH_MULTI_EVAL_MEAS_LIST_SEM_MARGIN_AREA_POSITIVE_MINIMUM_RESULTS", "Descriptive Name"="Fetch Multi Eval Meas List SEM Margin Area Positive Minimum Results", "Data Type"=enum."RawString", "Command"="FETC:NRS:MEAS{instance}:MEV:LIST:SEM:MARG:AREA{Area}:POS:MIN?", "Access"=enum."Read Only", "Range Table"="", "Read Callback"="", "Write Callback"="", "Range Callback"="", "Check Callback"="", "Rngtable Callback"="", "Coerce Callback"="", "Supported Models"="", "Instrument Options"="", "Check Status Callback"="", "Flags"=0, "Help"="Return spectrum emission mask margin positions for all measured list mode segments. The results of the maximum trace (resulting in minimum margins) for positive offset frequencies are returned.\n\nThe results are returned as pairs per segment: <Reliability>, {<MarginPosX>, <MarginPosY>}seg 1, {<MarginPosX>, <MarginPosY>}seg 2, ...\n\nReturn values:  \n<Reliability>\n decimal\n\n<MarginPosX>\n float\nX-position of margin for selected area\nDefault unit:  Hz \n\n<MarginPosY>\n float\nY-position of margin for selected area\nDefault unit:  dB\n\nAvailable Repeated Capabilities:\ninstance: i0, i1, i2, i3, i4, i5, i6, i7, i8, i9, i10, i11, i12, i13, i14, i15, i16, i17, i18, i19, i20, i21, i22, i23, i24, i25, i26, i27, i28, i29, i30, i31, i32\r\nArea: a1, a2, a3, a4, a5, a6, a7, a8, a9, a10, a11, a12\r\n\nRemote-control command(s):\nFETCh:NRSub:MEAS<i>:MEValuation:LIST:SEMask:MARGin:AREA<no>:POSitiv:MINimum?"}, {"Level"=6, "Class Only"=FALSE, "Identifier"="RSCMWXPNRFR1M_ATTR_FETCH_MULTI_EVAL_MEAS_LIST_SEM_MARGIN_AREA_NEGATIVE_CURRENT_RESULTS", "Descriptive Name"="Fetch Multi Eval Meas List SEM Margin Area Negative Current Results", "Data Type"=enum."RawString", "Command"="FETC:NRS:MEAS{instance}:MEV:LIST:SEM:MARG:AREA{Area}:NEG:CURR?", "Access"=enum."Read Only", "Range Table"="", "Read Callback"="", "Write Callback"="", "Range Callback"="", "Check Callback"="", "Rngtable Callback"="", "Coerce Callback"="", "Supported Models"="", "Instrument Options"="", "Check Status Callback"="", "Flags"=0, "Help"="Return spectrum emission mask margin positions for all measured list mode segments. The results of the current trace for negative offset frequencies are returned.\n\nThe results are returned as pairs per segment: <Reliability>, {<MarginPosX>, <MarginPosY>}seg 1, {<MarginPosX>, <MarginPosY>}seg 2, ...\n\nReturn values:  \n<Reliability>\n decimal\n\n<MarginPosX>\n float\nX-position 
